vi "Set DI Settings by DI TaskName in Dict.vi"(8 "error in (no error)":errorcluster, 9 "DI Settings":T1, 10 "DI TaskName":string, 11 "DAQ":refnum<class "DAQ.lvclass">) -> (0 "error out":errorcluster, 1 "DI Settings":T1, 3 "DAQ":refnum<class "DAQ.lvclass">)   [LabVIEW 2017, in "DAQ.lvclass"]
doc: "Developed by Kevin Thompson\nkevin@thompsonengineering.net\n\nCopyright 2018-2020\nThompson Engineering, LLC"
uses:
  DAQ.lvclass
  DataTypes/TD DI Instrument Settings--cluster.ctl
  DAQ.lvclass/DAQ.ctl
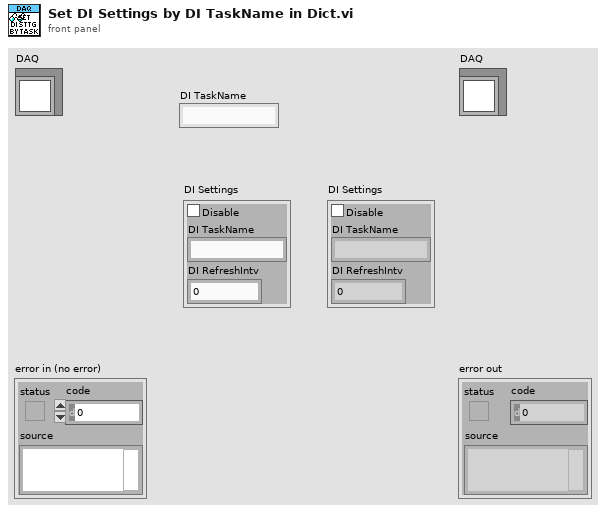
[diagram p1: front panel]
types:
  T1 = typedef "DAQ.lvclass/TD DI Instrument Settings--cluster.ctl" = cluster{"Disable":bool, "DI TaskName":string, "DI RefreshIntv":i32}
  T2 = typedef "TD Dynamic CVT DVR--ref.ctl" = refnum<data-value>
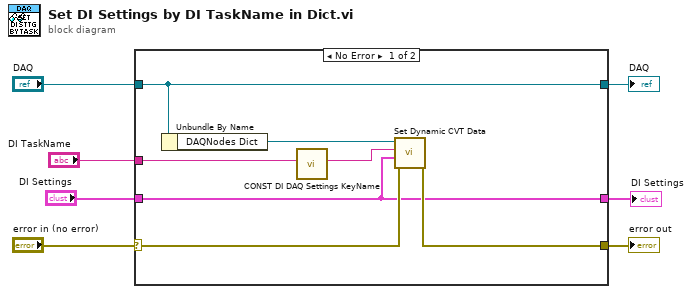
[diagram p0: block diagram]
diagram:
  n1 = case shown="No Error" "error in (no error)" {
    selector: "error in (no error)" -> [w11 w16]
    tunnel: [w9 w16] -> w6
    tunnel: [w14 w17] -> w4
    tunnel: "DAQ" -> [w14 w17]
    tunnel: "DI TaskName" -> [w13 _]
    tunnel: "DI Settings" -> [w8 w15]
    tunnel: [w8 w15] -> w1
    frame No Error {
      n2 = Unbundle By Name(w14) -> ("DAQNodes Dict"=w12:T2)
      n3 = call "CONST DI DAQ Settings KeyName.vi"("DI TaskName"=w13) -> ("DI DAQ Settings (KeyName)"=w10:string)  [unwired: 10 in]
      n4 = call <vilib>:"Set Dynamic CVT Data.vi"("error in (no error)"=w11, "value"=w8, "DataName"=w10, "dCVT DVR"=w12) -> ("error out"=w9:errorcluster)  [unwired: 5 in, 2 out]
    }
    frame Error {
    }
  }
  "error out" <- w6
  "DAQ" <- w4
  "DI Settings" <- w1
